vi "Update Authors Name.vi"(0 "INI File Ref In":T1, 1 "Config Data In":cluster{"Company":string, "Author":string}={"Company"="Good Automation, LLC", "Author"="Your Name Here"}, 3 "error in":errorcluster) -> (7 "INI File Ref Out":T1, 8 "Config Data Out":cluster{"Company":string, "Author":string}={"Company"="Good Automation, LLC", "Author"="Your Name Here"}, 10 "error out":errorcluster)   [LabVIEW 2014]
doc: "<b>VI Description:</b> This VI updates the author's name field in the INI file for the RCF Documentation Tool. \n<b>VI Version:</b> 1.0.23.beta \n<b>Review Date:</b> 03/09/2012 \n<b>Author:</b> Jason Willis, Ryan Podsim \n<b>Copyright:</b> Copyright © 2012-2014"
uses:
  <vilib>/Utility/config.llb/Config Data RefNum.ctl
  <vilib>/Utility/config.llb/Write Key (String).vi
  <vilib>/Utility/config.llb/NI_LVConfig.lvlib
panel:
  in  "Cancel":bool
  in  "Author's Name":string
  in  "Save":bool
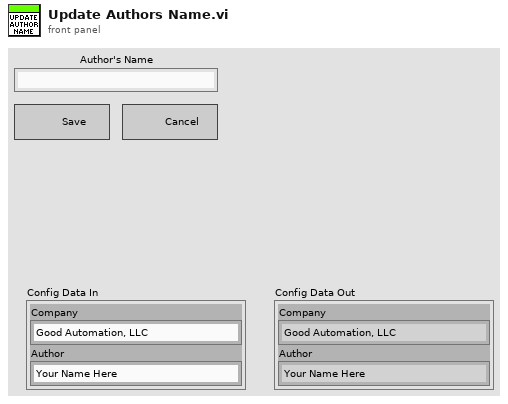
[diagram p1: front panel]
types:
  T1 = typedef "NI_LVConfig.lvlib/Config Data RefNum.ctl" = refnum<k1>
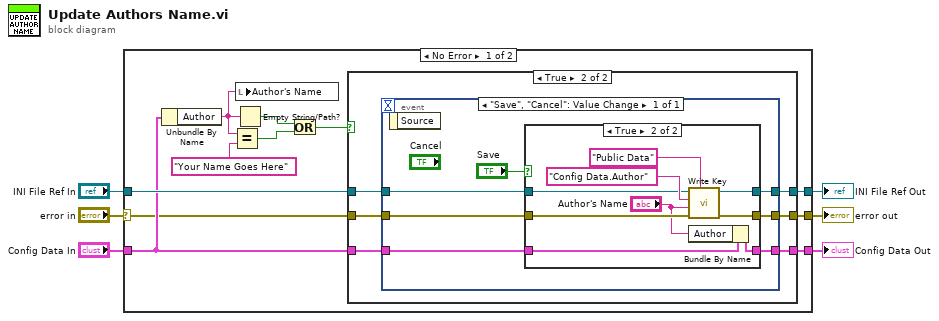
[diagram p0: block diagram]
diagram:
  n1 = case shown="No Error" "error in" {
    selector: "error in" -> [w7 w48]
    tunnel: [w12 w47] -> w6
    tunnel: "INI File Ref In" -> [w11 w47]
    tunnel: [w10 w46] -> w4
    tunnel: "Config Data In" -> [w9 w46]
    tunnel: [w8 w48] -> w2
    frame No Error {
      n2 = Unbundle By Name(w9) -> ("Author"=w14:string)
      n3 = Equal?(x=w14, y="Your Name Goes Here") -> (x = y?=w16:bool)
      n4 = Empty String/Path?(string/path=w14) -> (empty?=w17:bool)
      n5 = local write "Author's Name"(w14) -> ()
      n6 = Or(x=w17, y=w16) -> (x .or. y?=w13:bool)
      n7 = case shown="True" w13 {
        tunnel: [w20 w25] -> w12
        tunnel: w11 -> [w20 w26]
        tunnel: [w19 w21] -> w10
        tunnel: w9 -> [w19 w22]
        tunnel: w7 -> [w18 w24]
        tunnel: [w18 w23] -> w8
        frame False {
        }
        frame True {
          n8 = event shown="[0] \"Save\", \"Cancel\": Value Change" {
            selector: _ -> [_]
            dyn-events: _ -> [_]
            timeout: _ -> [_]
            tunnel: w26 -> [w33]
            tunnel: [w32] -> w25
            tunnel: w24 -> [w31]
            tunnel: [w30] -> w23
            tunnel: w22 -> [w28]
            tunnel: [w27] -> w21
            event "Save", "Cancel": Value Change {
              n9 = event-data() -> ()  [unwired: 1 in, 1 out]
              n10 = case shown="True" "Save" {
                tunnel: w33 -> [w36 w43]
                tunnel: [w36 w42] -> w32
                tunnel: w31 -> [w35 w41]
                tunnel: [w35 w40] -> w30
                tunnel: w28 -> [w34 w39]
                tunnel: [w34 w38] -> w27
                frame False {
                }
                frame True {
                  n11 = call-poly <vilib>:"Write Key.vi"("section"="Public Data" ("Section"), "error in (no error)"=w41, "value"="Author's Name", "key"="Config Data.Author" ("Key"), "refnum"=w43) -> ("error out"=w40:errorcluster, "refnum out"=w42:T1)  [unwired: 4 in, 1 out]
                  n12 = Bundle By Name(cluster=w39, "Author"="Author's Name") -> (w38:cluster{"Company":string, "Author":string})
                }
              }
            }
          }
        }
      }
    }
    frame Error {
    }
  }
  "INI File Ref Out" <- w6
  "error out" <- w2
  "Config Data Out" <- w4
